vi "Write Multi Channel Data.vi"(8 "error in":errorcluster, 9 "Data":waveform(dbl)[](array[waveform]), 10 "Current Group":string, 11 "TDMS in":refnum<class "TDMS.lvclass">) -> (0 "error out":errorcluster, 3 "TDMS out":refnum<class "TDMS.lvclass">)   [LabVIEW 2019, in "TDMS.lvlib" / "TDMS.lvclass"]
uses:
  TDMS.lvclass
  TDMS.lvclass/TDMS.ctl
  Read TDMS Ref.vi
  Write TDMS Ref.vi
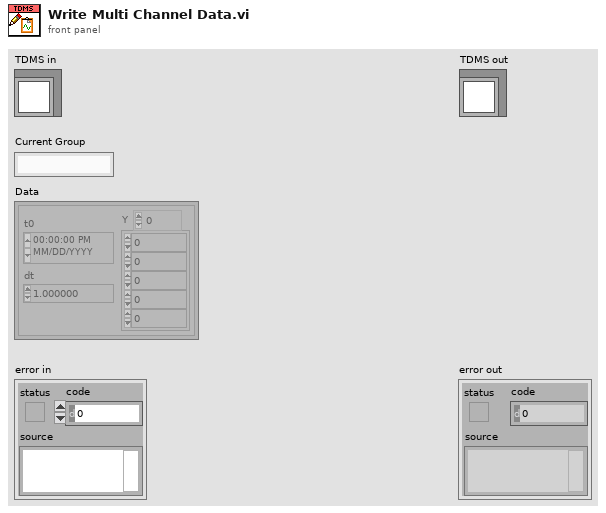
[diagram p1: front panel]
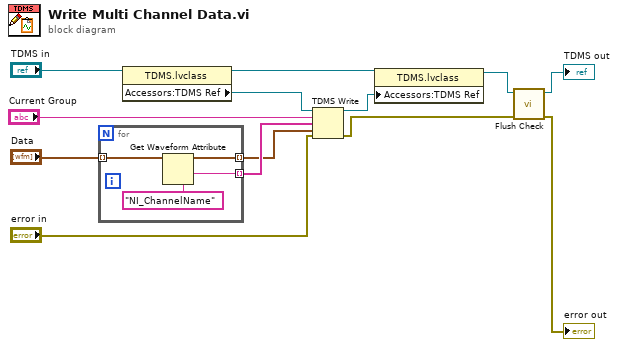
[diagram p0: block diagram]
diagram:
  n1 = for {
    tunnel: "Data" -> [w15] mode=indexing
    tunnel: [w16] -> w7 mode=indexing
    tunnel: [w14] -> w6 mode=indexing
    w17 = "NI_ChannelName" ("name")
    n2 = Get Waveform Attribute(5:w17, 6:w17, 7:w15) -> (1:w16:string, 3:w14:waveform(dbl))  [unwired: 1 in, 2 out]
  }
  n3 = property class="TDMS.lvclass"(reference="TDMS in") -> (reference out=w11:refnum<class "TDMS.lvclass">, "Accessors:TDMS Ref"=w12:refnum<k34>)  [unwired: 1 in, 1 out]
  n4 = TDMS Write(0:w12, 5:"Current Group", 7:w7, 9:w6, 11:"error in") -> (4:w10:refnum<k34>, 15:w3:errorcluster)  [unwired: 1 in, 2 out]
  n5 = property class="TDMS.lvclass"(reference=w11, "Accessors:TDMS Ref"=w10) -> (reference out=w5:refnum<class "TDMS.lvclass">)  [unwired: 1 in, 1 out]
  n6 = call "Flush Check.vi"("error in (no error)"=w3, "TDMS in"=w5) -> ("error out"=→"error out":errorcluster, "TDMS out"=→"TDMS out":refnum<class "TDMS.lvclass">)  [unwired: 8 in]
